vi "Remove Overflow FXP(+-,14,1)x8ch.vi"(4 "data in":T1={"channel 0"=[0.0, 0.0], "channel 1"=[0.0, 0.0], "channel 2"=[0.0, 0.0], "channel 3"=[0.0, 0.0], "channel 4"=[0.0, 0.0], "channel 5"=[0.0, 0.0], "channel 6"=[0.0, 0.0], "channel 7"=[0.0, 0.0]}) -> (0 "overflow":bool, 1 "data out":T1)   [LabVIEW 2014]
doc: "Removes and returns carried overflow from input data.\n\n<B>Supported data types</B>\nFXP +-,18,1; FXP +-,14,1\n\n<B>Supported channel size</B>\n4, 8\n\n<B>Supported samples per cycle</B>\n2\n\n<B>Input Parameters</B>\n\n<B>data in</B> specifies the data input carrying the overflow.\n\n<B>Output Parameters</B>\n\n<B>data out</B> returns the data without the overflow.\n\n<B>overflow</B> returns the overflow that was carried in the data input."
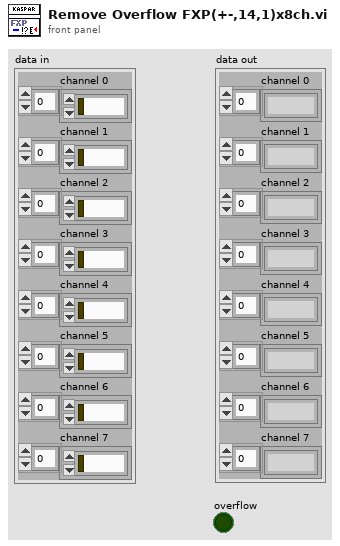
[diagram p1: front panel]
types:
  T1 = cluster{"channel 0":fxp<+/-,14,1>[], "channel 1":fxp<+/-,14,1>[], "channel 2":fxp<+/-,14,1>[], "channel 3":fxp<+/-,14,1>[], "channel 4":fxp<+/-,14,1>[], "channel 5":fxp<+/-,14,1>[], "channel 6":fxp<+/-,14,1>[], "channel 7":fxp<+/-,14,1>[]}
  T2 = cluster{"data out":fxp<+/-,14,1>[], "data out":fxp<+/-,14,1>[], "data out":fxp<+/-,14,1>[], "data out":fxp<+/-,14,1>[], "data out":fxp<+/-,14,1>[], "data out":fxp<+/-,14,1>[], "data out":fxp<+/-,14,1>[], "data out":fxp<+/-,14,1>[]}
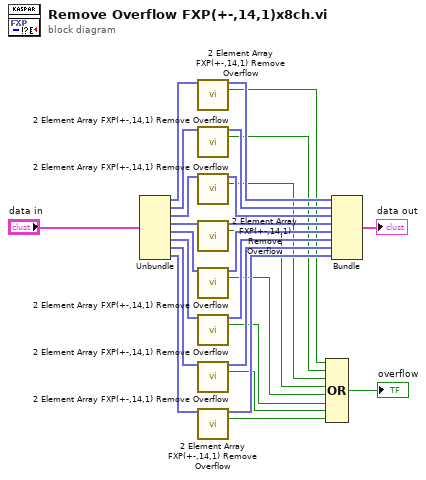
[diagram p0: block diagram]
diagram:
  n1 = Unbundle("data in") -> ("channel 0"=w25:fxp<+/-,14,1>[], "channel 1"=w23:fxp<+/-,14,1>[], "channel 2"=w21:fxp<+/-,14,1>[], "channel 3"=w19:fxp<+/-,14,1>[], "channel 4"=w17:fxp<+/-,14,1>[], "channel 5"=w11:fxp<+/-,14,1>[], "channel 6"=w13:fxp<+/-,14,1>[], "channel 7"=w15:fxp<+/-,14,1>[])
  n2 = call "2 Element Array FXP(+-,14,1) Remove Overflow.vi"("data in"=w25) -> ("data out"=w24:fxp<+/-,14,1>[], "overflow"=w9:bool)  [unwired: 13 in]
  n3 = call "2 Element Array FXP(+-,14,1) Remove Overflow.vi"("data in"=w23) -> ("data out"=w22:fxp<+/-,14,1>[], "overflow"=w8:bool)  [unwired: 13 in]
  n4 = call "2 Element Array FXP(+-,14,1) Remove Overflow.vi"("data in"=w21) -> ("data out"=w20:fxp<+/-,14,1>[], "overflow"=w7:bool)  [unwired: 13 in]
  n5 = call "2 Element Array FXP(+-,14,1) Remove Overflow.vi"("data in"=w19) -> ("data out"=w18:fxp<+/-,14,1>[], "overflow"=w6:bool)  [unwired: 13 in]
  n6 = call "2 Element Array FXP(+-,14,1) Remove Overflow.vi"("data in"=w17) -> ("data out"=w16:fxp<+/-,14,1>[], "overflow"=w5:bool)  [unwired: 13 in]
  n7 = call "2 Element Array FXP(+-,14,1) Remove Overflow.vi"("data in"=w11) -> ("data out"=w10:fxp<+/-,14,1>[], "overflow"=w4:bool)  [unwired: 13 in]
  n8 = call "2 Element Array FXP(+-,14,1) Remove Overflow.vi"("data in"=w13) -> ("data out"=w12:fxp<+/-,14,1>[], "overflow"=w3:bool)  [unwired: 13 in]
  n9 = call "2 Element Array FXP(+-,14,1) Remove Overflow.vi"("data in"=w15) -> ("data out"=w14:fxp<+/-,14,1>[], "overflow"=w2:bool)  [unwired: 13 in]
  n10 = Compound Arithmetic op=OR(w9, w8, w7, w6, w5, w4, w3, w2) -> (→"overflow":bool)
  n11 = Bundle("data out"=w24, "data out"=w22, "data out"=w20, "data out"=w18, "data out"=w16, "data out"=w10, "data out"=w12, "data out"=w14) -> (→"data out":T2)  [unwired: 1 in]
